vi "Calculate Test Gaps.vi"(10 "VIs Without Test Coverage by path":path[](array[path])) -> (1 "folder names":string[](array[string]), 2 "% of gap values":dbl[](array[numeric]))   [LabVIEW 2009, in "GraphicalTestRunner.lvlib"]
uses:
  Graphical Test Runner/Graphical Test Runner Support/GraphicalTestRunner.lvlib
  <userlib>/_OpenG.lib/array/array.llb/Remove Duplicates from 1D Array (Path)__ogtk.vi
  <userlib>/_OpenG.lib/file/file.llb/Strip Path - Arrays__ogtk.vi
  <userlib>/_OpenG.lib/array/array.llb/Search 1D Array (Path)__ogtk.vi
  <userlib>/_OpenG.lib/file/file.llb/Strip Path - Traditional__ogtk.vi
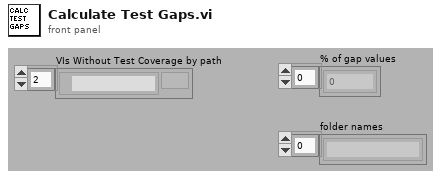
[diagram p1: front panel]
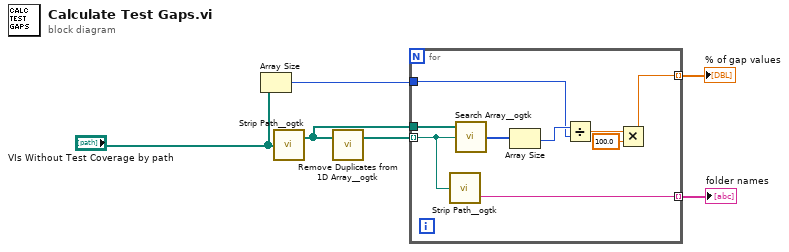
[diagram p0: block diagram]
diagram:
  n1 = Array Size(array="VIs Without Test Coverage by path") -> (size(s)=w4:i32)
  n2 = call-poly <userlib>:"Strip Path__ogtk.vi"("path"="VIs Without Test Coverage by path") -> ("stripped path"=w1:path[])  [unwired: 1 out]
  n3 = call-poly <userlib>:"Remove Duplicates from 1D Array__ogtk.vi"("Input Array"=w1) -> ("Output Array"=w6:path[])  [unwired: 1 out]
  n4 = for {
    tunnel: w6 -> [w8] mode=indexing
    tunnel: w1 -> [w15]
    tunnel: w4 -> [w12]
    tunnel: [w9] -> w3 mode=indexing
    tunnel: [w7] -> w2 mode=indexing
    n5 = call-poly <userlib>:"Strip Path__ogtk.vi"("path"=w8) -> ("name"=w7:string)  [unwired: 1 out]
    n6 = call-poly <userlib>:"Search Array__ogtk.vi"("Array"=w15, "Element Data"=w8) -> ("Indices of Elements"=w14:i32[])  [unwired: 7 in]
    n7 = Array Size(array=w14) -> (size(s)=w13:i32)
    n8 = Divide(x=w13, y=w12) -> (x/y=w11:dbl)
    n9 = Multiply(x=w11, y=100.0) -> (x*y=w9:dbl)
  }
  "folder names" <- w2
  "% of gap values" <- w3
